vi "Select Actor Dialog.vi"(8 "Error In":errorcluster, 11 "CS++StartActor in":refnum<class "CS++StartActor.lvclass">) -> (0 "Error Out":errorcluster, 2 "Selected Names":string[](array[string]), 3 "CS++StartActor out":refnum<class "CS++StartActor.lvclass">)   [LabVIEW 2013, in "CS++StartActor.lvlib" / "CS++StartActor.lvclass"]
doc: "Read Actor List from DB and display selection dialog."
uses:
  CS++StartActor.lvclass
  CS++StartActor.lvclass/CS++StartActor.ctl
panel:
  in  "Actor List":i32[](listbox)
  in  "Cancel":bool
  in  "Launch":bool
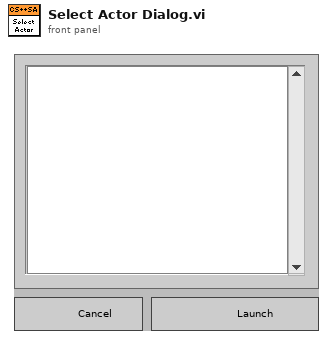
[diagram p1: front panel]
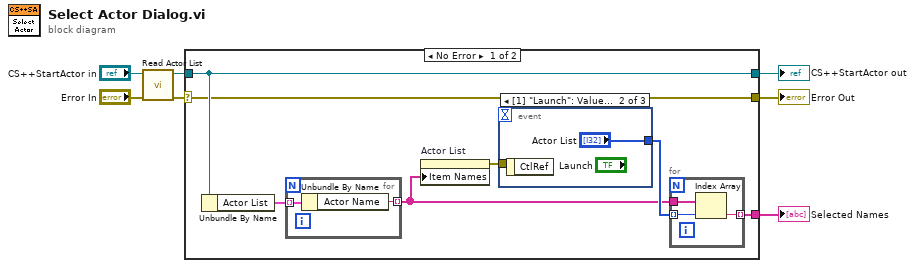
[diagram p0: block diagram]
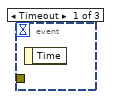
[diagram p2: hidden frame]
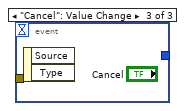
[diagram p3: hidden frame]
diagram:
  n1 = call "Read Actor List.vi"("error in (no error)"="Error In", "CS++StartActor in"="CS++StartActor in") -> ("error out"=w4:errorcluster, "CS++StartActor out"=w5:refnum<class "CS++StartActor.lvclass">)  [unwired: 8 in]
  n2 = case shown="No Error" w4 {
    selector: w4 -> [w8 w21]
    tunnel: [w12 _] -> w7
    tunnel: w5 -> [w9 w22]
    tunnel: [w9 w22] -> w3
    tunnel: [w8 w21] -> w1
    frame No Error {
      n3 = Unbundle By Name(w9) -> ("Actor List"=w10:cluster{"Actor Name":string, "Open":bool}[])
      n4 = for {
        tunnel: w10 -> [w16] mode=indexing
        tunnel: [w15] -> w11 mode=indexing
        n5 = Unbundle By Name(w16) -> ("Actor Name"=w15:string)
      }
      n6 = property on="Actor List" class="LstBox (strict)"("Item Names"=w11) -> (error out=w14:errorcluster)  [unwired: 2 in, 1 out]
      n7 = event shown="[1] \"Launch\": Value Change;  \"Actor List\": Double Click" {
        selector: _ -> [_ _ _]
        dyn-events: _ -> [_ _ _]
        timeout: _ -> [_ _ _]
        tunnel: [_ "Actor List" _] -> w13
        tunnel: w14 -> [_ _ _]
        event Timeout {
          n8 = event-data() -> ()  [unwired: 1 in, 1 out]
        }
        event "Launch": Value Change; "Actor List": Double Click {
          n9 = event-data() -> ()  [unwired: 1 in, 1 out]
        }
        event "Cancel": Value Change {
          n10 = event-data() -> ()  [unwired: 1 in, 2 out]
        }
      }
      n11 = for {
        tunnel: w13 -> [w18] mode=indexing
        tunnel: w11 -> [w19]
        tunnel: [w17] -> w12 mode=indexing
        n12 = Index Array(array=w19, index=w18) -> (element=w17:string)
      }
    }
    frame Error {
    }
  }
  "Selected Names" <- w7
  "CS++StartActor out" <- w3
  "Error Out" <- w1
